vi "main.vi"() -> ()   [LabVIEW 2011]
uses:
  <vilib>/userDefined/High Color/IMAQdx.ctl
  global_vars.vi
  <vilib>/vision/driver/NI_Vision_Acquisition_Software.lvlib
panel:
  in  "b_default prefix":bool
  in  "ID_Camera":T1="cam0" caption="Camera in Use"
  in  "b_orig":bool caption="original"
  in  "b_captured":bool caption="captured"
  in  "image prefix":string
  out "b_meas_running":bool caption="Measurement\nRunning"
  in  "Color":u32(colorbox)=16448250
  in  "b_preview fringes":bool
  in  "df_intial phase shift":dbl
  in  "b_record images":bool
  in  "UL_#Phase Shifts":i32=4
  out "p_experiment_path":path=path "X:/Cloud Drives/Dropbox/Europhotonics/FringeMan/Image Storage/01_23"
  in  "EXP File Path 2":path=path "C:/Users/ccquiel/Dropbox/Personal Project/Image Storage/Unwrapped Phase Maps" caption="Enter or select file path"
  in  "b_save images":bool caption="save images"
  in  "b_start_meas":bool
  in  "center radius":dbl
  in  "b_align":bool
  in  "number of rings":i32=20
  in  "df_#fringes":dbl=4.0 caption="#fringes"
  in  "fullscreen?":bool
  in  "to second \nscreen?":bool
  in  "floating":bool=TRUE
  in  "title bar":bool=TRUE
  in  "y height(Px)":i32=500
  in  "x Width(Px)":i32=1000
  in  "Stop Button":bool
  # "Window Control"
  # "Alignment Control"
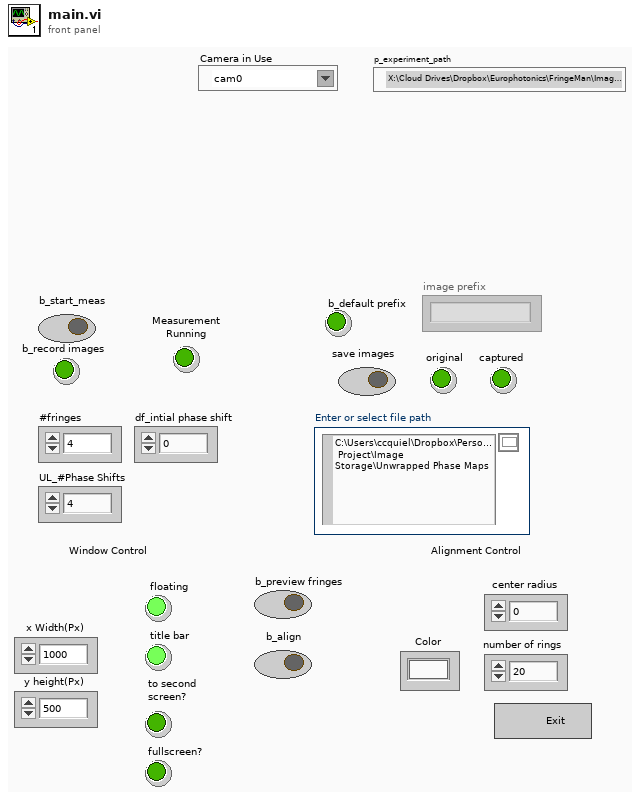
[diagram p1: front panel]
types:
  T1 = typedef "IMAQdx.ctl" = refnum<k21>
  T2 = enum8{"Enabled", "Disabled", "Disabled and Grayed Out"}
  T3 = typedef "IMAQ Image.ctl" = refnum<image>
  T4 = cluster{"Numeric Control":i16, "Numeric Control":i16}
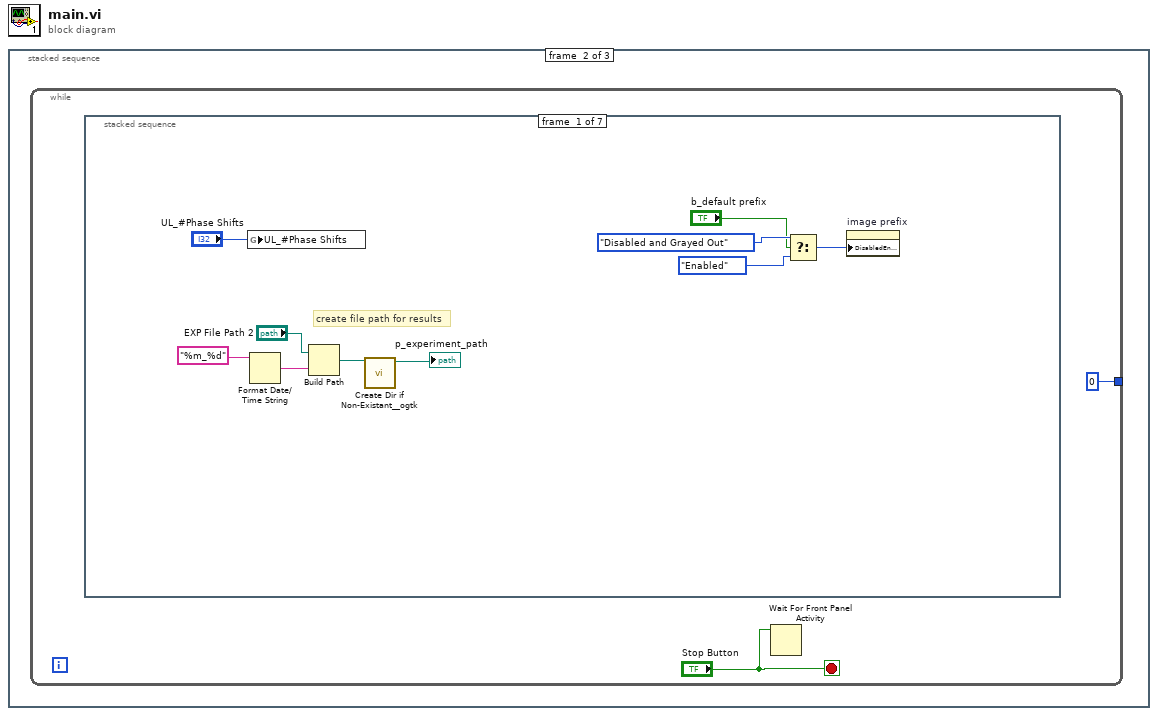
[diagram p0: block diagram]
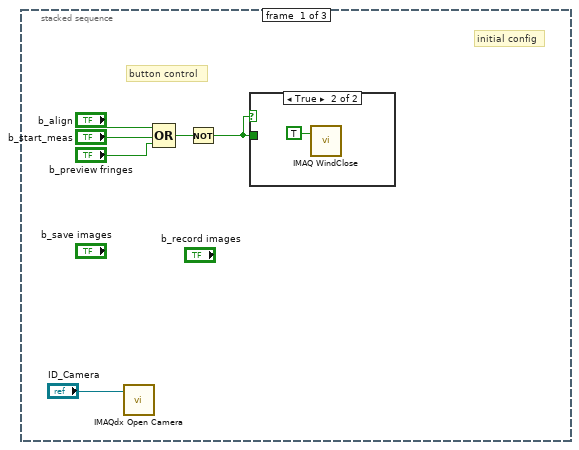
[diagram p2: hidden frame]
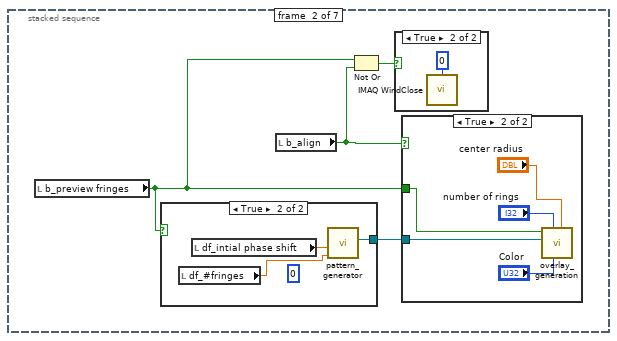
[diagram p4: hidden frame]
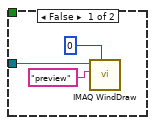
[diagram p6: hidden frame]
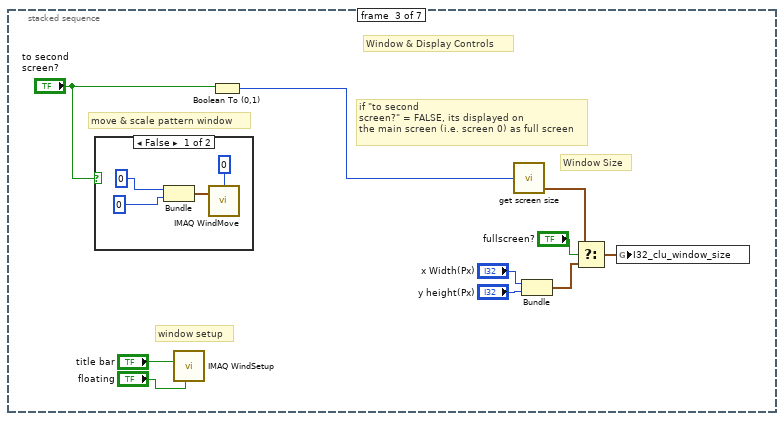
[diagram p8: hidden frame]
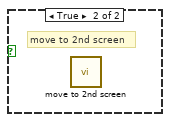
[diagram p9: hidden frame]
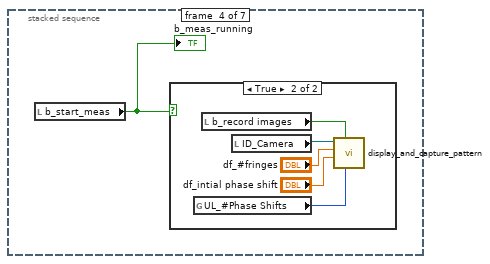
[diagram p10: hidden frame]
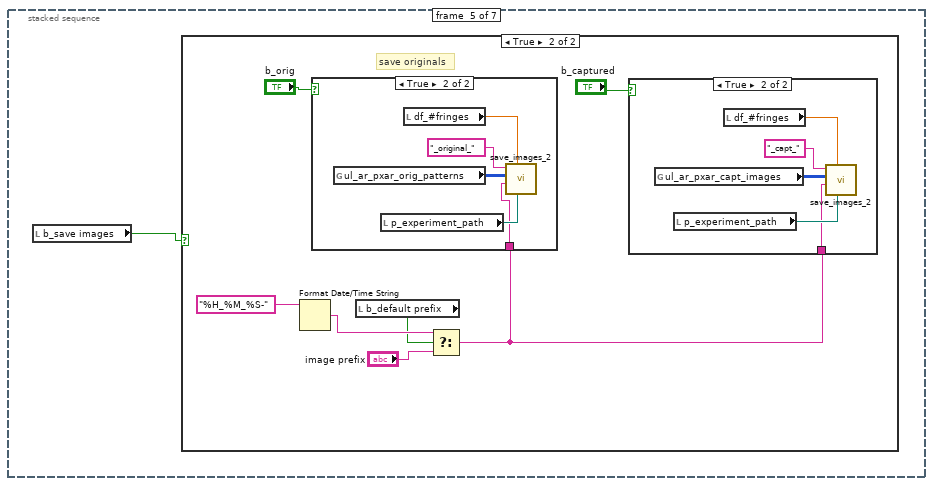
[diagram p12: hidden frame]
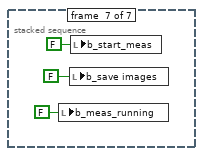
[diagram p17: hidden frame]
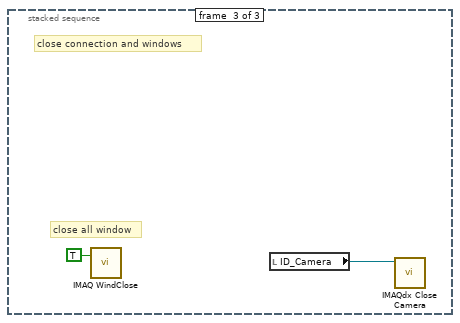
[diagram p18: hidden frame]
diagram:
  n1 = stacked-sequence {
    frame #0 {
      # "initial config"
      # "button control"
      n2 = call <vilib>:"IMAQdx Open Camera.vi"("Session In"="ID_Camera") -> ()  [unwired: 9 in, 2 out]
      n3 = Compound Arithmetic op=OR("b_align", "b_start_meas", "b_preview fringes") -> (w2:bool)
      n4 = Not(x=w2) -> (.not. x?=w1:bool)
      n5 = case shown="True" w1 {
        tunnel: w1 -> [_ _]
        frame False {
        }
        frame True {
          n6 = call "IMAQ WindClose"("Close All Windows (False)"=TRUE) -> ()  [unwired: 5 in, 1 out]
        }
      }
    }
    frame #1 {
      n7 = while {
        tunnel: [0] -> _
        stop <- "Stop Button" stop-if-true
        n8 = stacked-sequence {
          frame #0 {
            # "create file path for results"
            n9 = global write "global_vars.vi" "UL_#Phase Shifts"("UL_#Phase Shifts") -> ()
            n10 = Format Date/Time String(time format string (%c)="%m_%d") -> (date/time string=w16:string)  [unwired: 2 in]
            n11 = Build Path(base path="EXP File Path 2", name or relative path=w16) -> (appended path=w15:path)
            n12 = call <userlib>:"Create Dir if Non-Existant__ogtk.vi"("Directory Path"=w15) -> ("dup Directory Path"=→"p_experiment_path":path)  [unwired: 8 in, 2 out]
            n13 = Select(t=T2."Disabled and Grayed Out" ("Disabled"), s="b_default prefix", f=T2."Enabled" ("Disabled")) -> (s? t:f=w10:T2)
            n14 = property on="image prefix" class="Str"("DisabledEnum"=w10) -> ()  [unwired: 2 in, 2 out]
          }
          frame #1 {
            n15 = local read "b_preview fringes"() -> (w20:bool)
            n16 = case shown="True" w20 {
              tunnel: [_ w33] -> w23
              frame False {
              }
              frame True {
                (unwired) 0 ("Window Number (0...15)")
                n17 = local read "df_#fringes"() -> (w35:dbl)
                n18 = local read "df_intial phase shift"() -> (w34:dbl)
                n19 = call "pattern_generator.vi"("fringe number"=w35, "phase"=w34) -> ("fringe pattern"=w33:T3)  [unwired: 8 in, 1 out]
              }
            }
            n20 = local read "b_align"() -> (w21:bool)
            n21 = Not Or(1:w21, 2:w20) -> (0:w22:bool)
            n22 = case shown="True" w22 {
              frame False {
              }
              frame True {
                n23 = call "IMAQ WindClose"("Window Number (0...15)"=0) -> ()  [unwired: 5 in, 1 out]
              }
            }
            n24 = case shown="True" w21 {
              tunnel: w23 -> [w26 w30]
              tunnel: w20 -> [_ w29]
              frame False {
                n25 = call "IMAQ WindDraw"("Window Number (0...15)"=0, "Title"="preview", "Image"=w26) -> ()  [unwired: 7 in, 2 out]
              }
              frame True {
                n26 = call "overlay_generation.vi"("center radius"="center radius", "Color"="Color", "number of rings"="number of rings", "Image Src"=w30, "fringe preview on"=w29) -> ()  [unwired: 7 in]
              }
            }
          }
          frame #2 {
            # "if \"to second \nscreen?\" = FALSE, its displayed on \nthe main screen (i.e. screen 0) as full screen"
            # "Window Size"
            # "Window & Display Controls"
            # "window setup"
            # "move & scale pattern window"
            n27 = case shown="False" "to second \nscreen?" {
              frame False {
                n28 = Bundle(0, 0) -> (w49:cluster{i32, i32})  [unwired: 1 in]
                n29 = call "IMAQ WindMove"("Window Number (0...15)"=0, "Coordinates (screen)"=w49) -> ()  [unwired: 3 in, 2 out]
              }
              frame True {
                # "move to 2nd screen"
                n30 = call "move to 2nd screen.vi"() -> ()  [unwired: 12 in]
              }
            }
            n31 = call "IMAQ WindSetup"("Window is floating? (No)"="floating", "Window has title bar? (Yes)"="title bar") -> ()  [unwired: 9 in, 1 out]
            n32 = Boolean To (0,1)(Boolean="to second \nscreen?") -> (0, 1=w36:i16)
            n33 = call "get screen size.vi"("screen"=w36) -> ("wind size (width/height)"=w38:T4)  [unwired: 2 in, 2 out]
            n34 = Bundle("x Width(Px)"="x Width(Px)", "y height(Px)"="y height(Px)") -> (w40:cluster{"x Width(Px)":i32, "y height(Px)":i32})  [unwired: 1 in]
            n35 = Select(t=w38, s="fullscreen?", f=w40) -> (s? t:f=w39:cluster{"x Width(Px)":i32, "y height(Px)":i32})
            n36 = global write "global_vars.vi" "I32_clu_window_size"(w39) -> ()
          }
          frame #3 {
            n37 = local read "b_start_meas"() -> (w50:bool)
            "b_meas_running" <- w50
            n38 = case shown="True" w50 {
              frame False {
              }
              frame True {
                n39 = global read "global_vars.vi" "UL_#Phase Shifts"() -> (w55:i32)
                n40 = local read "b_record images"() -> (w52:bool)
                n41 = local read "ID_Camera"() -> (w51:T1)
                n42 = call "display_and_capture_pattern.vi"("#Phase Shifts"=w55, "capture images ?"=w52, "intial phase shift"="df_intial phase shift", "#fringes"="df_#fringes", "Camera ID"=w51) -> ()  [unwired: 7 in]
              }
            }
          }
          frame #4 {
            n43 = local read "b_save images"() -> (w56:bool)
            n44 = case shown="True" w56 {
              frame False {
              }
              frame True {
                # "save originals"
                n45 = Format Date/Time String(time format string (%c)="%H_%M_%S-") -> (date/time string=w62:string)  [unwired: 2 in]
                n46 = local read "b_default prefix"() -> (w57:bool)
                n47 = Select(t=w62, s=w57, f="image prefix") -> (s? t:f=w60:string)
                n48 = case shown="True" "b_orig" {
                  tunnel: w60 -> [_ w69]
                  frame False {
                  }
                  frame True {
                    n49 = global read "global_vars.vi" "ul_ar_pxar_orig_patterns"() -> (w70:u8[][][])
                    n50 = local read "p_experiment_path"() -> (w72:path)
                    n51 = local read "df_#fringes"() -> (w73:dbl)
                    n52 = call "save_images_2.vi"("p_experiment_path"=w72, "number of fringes"=w73, "time (or other uniqe identifier)"=w69, "images to store (3D pixel array)"=w70, "description (orig./capt.)"="_original_") -> ()  [unwired: 7 in]
                  }
                }
                n53 = case shown="True" "b_captured" {
                  tunnel: w60 -> [_ w64]
                  frame False {
                  }
                  frame True {
                    n54 = global read "global_vars.vi" "ul_ar_pxar_capt_images"() -> (w65:u8[][][])
                    n55 = local read "p_experiment_path"() -> (w67:path)
                    n56 = local read "df_#fringes"() -> (w68:dbl)
                    n57 = call "save_images_2.vi"("p_experiment_path"=w67, "number of fringes"=w68, "time (or other uniqe identifier)"=w64, "images to store (3D pixel array)"=w65, "description (orig./capt.)"="_capt_") -> ()  [unwired: 7 in]
                  }
                }
              }
            }
          }
          frame #5 {
            # "this is all yours ccquiel"
            # "calc. phase maps"
          }
          frame #6 {
            n58 = local write "b_meas_running"(FALSE ("b_meas_running")) -> ()
            n59 = local write "b_save images"(FALSE ("b_save images")) -> ()
            n60 = local write "b_start_meas"(FALSE ("b_start_meas")) -> ()
          }
        }
        n61 = Wait For Front Panel Activity(3:"Stop Button") -> ()  [unwired: 2 in, 1 out]
      }
    }
    frame #2 {
      # "close connection and windows"
      # "close all window"
      n62 = call "IMAQ WindClose"("Close All Windows (False)"=TRUE) -> ()  [unwired: 5 in, 1 out]
      n63 = local read "ID_Camera"() -> (w77:T1)
      n64 = call <vilib>:"IMAQdx Close Camera.vi"("Session In"=w77) -> ()  [unwired: 10 in, 1 out]
    }
  }
